vi "SP Fill Limit With NaN.vi"(7 "Number of Points":i32, 11 "Limit":dbl[](array[numeric])) -> (3 "Filled Limit":dbl[](array[numeric]))   [LabVIEW 2011]
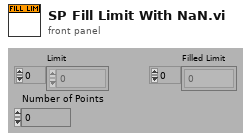
[diagram p1: front panel]
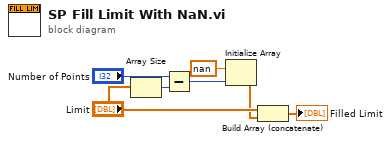
[diagram p0: block diagram]
diagram:
  n1 = Array Size(array="Limit") -> (size(s)=w7:i32)
  n2 = Subtract(x="Number of Points", y=w7) -> (x-y=w4:i32)
  n3 = Initialize Array(nan, w4) -> (w2:dbl[])
  n4 = Build Array (concatenate)("Limit", w2) -> (→"Filled Limit":dbl[])
